vi "PAN_RunMacro.vi"(8 "error in (no error)":errorcluster, 10 "commands":string, 11 "macrodir":path) -> (0 "error out":errorcluster, 2 "response":string)   [LabVIEW 2016]
panel:
  in  "type specifier VI Refnum (for type only)":refnum<vi>
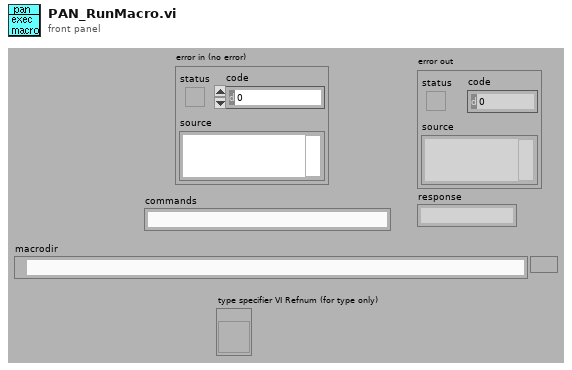
[diagram p1: front panel]
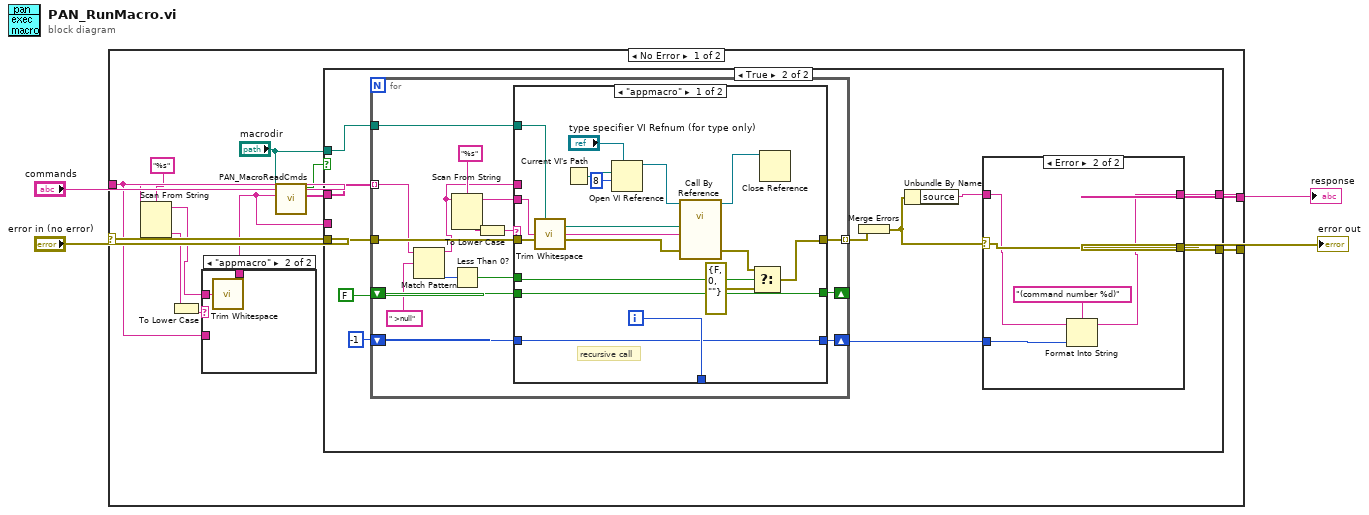
[diagram p0: block diagram]
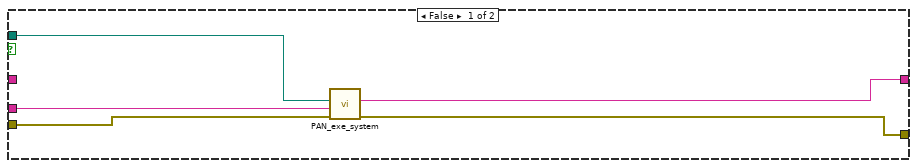
[diagram p3: hidden frame]
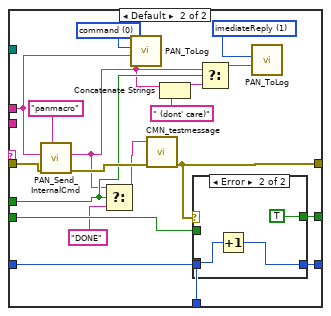
[diagram p5: hidden frame]
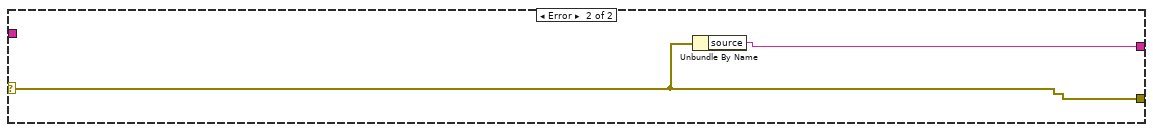
[diagram p7: hidden frame]
diagram:
  n1 = case shown="No Error" "error in (no error)" {
    selector: "error in (no error)" -> [w16 w99]
    tunnel: "commands" -> [w6 _]
    tunnel: [w14 w99] -> w3
    tunnel: [w15 w100] -> w2
    frame No Error {
      n2 = Scan From String(format string="%s", input string=w6) -> (remaining string=w7:string, output 1=w9:string)  [unwired: 2 in, 3 out]
      n3 = To Lower Case(string=w9) -> (all lower case string=w8:string)
      n4 = case shown="\"appmacro\"" w8 {
        tunnel: w7 -> [_ w19]
        tunnel: w6 -> [w17 _]
        tunnel: [w17 w18] -> w5
        frame Default {
        }
        frame "appmacro" {
          n5 = call <vilib>:"Trim Whitespace.vi"("string"=w19) -> ("trimmed string"=w18:string)  [unwired: 1 in]
        }
      }
      n6 = call "PAN_MacroReadCmds.vi"("CommandStr"=w5, "macrodir"="macrodir") -> ("commands"=w13:string[], "macro"=w12:bool)  [unwired: 8 out]
      n7 = case shown="True" w12 {
        tunnel: w16 -> [w22 w34]
        tunnel: [w21 w31] -> w15
        tunnel: [w20 w30] -> w14
        tunnel: w13 -> [_ w26]
        tunnel: "macrodir" -> [w24 w25]
        tunnel: w5 -> [w23 _]
        frame False {
          n8 = call "PAN_exe_system.vi"("error in (no error)"=w22, "command line"=w23, "working directory"=w24) -> ("error out"=w20:errorcluster, "response"=w21:string)  [unwired: 1 in, 6 out]
        }
        frame True {
          n9 = for {
            tunnel: w26 -> [w44] mode=indexing
            tunnel: [w56] -> w35 mode=indexing
            tunnel: w34 -> [w59]
            shift-right: [w54] -> _
            shift-left: FALSE -> [w53]
            shift-right: [w55] -> w27
            shift-left: -1 ("f") -> [w57]
            tunnel: w25 -> [w49]
            i -> [w58]
            n10 = Match Pattern(string=w44, regular expression=" >null") -> (before substring=w43:string, offset past match=w46:i32)  [unwired: 3 out]
            n11 = Scan From String(format string="%s", input string=w43) -> (remaining string=w48:string, output 1=w51:string)  [unwired: 2 in, 3 out]
            n12 = Less Than 0?(x=w46) -> (x < 0?=w45:bool)
            n13 = To Lower Case(string=w51) -> (all lower case string=w50:string)
            n14 = case shown="\"appmacro\"" w50 {
              tunnel: w59 -> [w69 w93]
              tunnel: w58 -> [_ w92]
              tunnel: w57 -> [w74 w91]
              tunnel: [w61 w90] -> w56
              tunnel: [w74 w89] -> w55
              tunnel: [w73 w88] -> w54
              tunnel: w53 -> [w73 w87]
              tunnel: w43 -> [_ w82]
              tunnel: w49 -> [w70 _]
              tunnel: w48 -> [w66 _]
              tunnel: w45 -> [w63 w79]
              frame "appmacro" {
                # "recursive call"
                n15 = call <vilib>:"Trim Whitespace.vi"("string"=w66) -> ("trimmed string"=w67:string)  [unwired: 1 in]
                n16 = Current VI's Path() -> (path=w68:path)
                n17 = Open VI Reference(type specifier VI Refnum (for type only)="type specifier VI Refnum (for type only)", vi path=w68, options=8) -> (vi reference=w71:refnum<vi>)  [unwired: 1 in, 3 out]
                n18 = call-by-ref "?"(reference=w71, "error in"=w69, "CommandStr"=w67, "macrodir"=w70) -> (reference out=w65:refnum<vi>, "error out"=w62:errorcluster)  [unwired: 8 in, 2 out]
                n19 = Select(t=w62, s=w63, f=errorcluster {"status"=FALSE, "code"=0, "source"=""}) -> (s? t:f=w61:errorcluster)
                n20 = Close Reference(reference=w65) -> ()  [unwired: 1 in, 1 out]
              }
              frame Default {
                w84 = u16 1 items=["command", "imediateReply", "Callback Reply", "Information"] ("type")
                w85 = u16 0 items=["command", "imediateReply", "Callback Reply", "Information"] ("type")
                n21 = call "PAN_Send_InternalCmd.vi"("taskID"="panmacro", "error in (no error)"=w93, "command"=w82) -> ("error out"=w86:errorcluster, "response"=w78:string)  [unwired: 2 in, 5 out]
                n22 = Select(t=w78, s=w79, f="DONE") -> (s? t:f=w81:string)
                n23 = call "PAN_ToLog.vi"("message"=w82, "type"=w85) -> ()  [unwired: 2 in, 8 out]
                n24 = call "CMN_testmessage.vi"("error in (no error)"=w86, "message  in"=w81) -> ("error out"=w90:errorcluster)  [unwired: 9 out]
                n25 = Concatenate Strings(w78, " (dont' care)" ("string")) -> (w76:string)
                n26 = case shown="Error" w90 {
                  tunnel: w92 -> [_ w97]
                  tunnel: w91 -> [w95 _]
                  tunnel: [w95 w96] -> w89
                  tunnel: [w94 TRUE] -> w88
                  tunnel: w87 -> [w94 _]
                  frame No Error {
                  }
                  frame Error {
                    n27 = Increment(x=w97) -> (x+1=w96:i32)
                  }
                }
                n28 = Select(t=w78, s=w79, f=w76) -> (s? t:f=w75:string)
                n29 = call "PAN_ToLog.vi"("message"=w75, "type"=w84) -> ()  [unwired: 2 in, 8 out]
              }
            }
          }
          n30 = Merge Errors(w35) -> (w33:errorcluster)
          n31 = Unbundle By Name(w33) -> ("source"=w32:string)
          n32 = case shown="Error" w33 {
            selector: w33 -> [w36 w42]
            tunnel: w32 -> [w37 w39]
            tunnel: [w37 w38] -> w31
            tunnel: [w36 w42] -> w30
            tunnel: w27 -> [_ w40]
            frame No Error {
            }
            frame Error {
              n33 = Format Into String(format string="(command number %d)", initial string=w39, w40) -> (resulting string=w38:string)  [unwired: 1 in, 1 out]
            }
          }
        }
      }
    }
    frame Error {
      n34 = Unbundle By Name(w99) -> ("source"=w100:string)
    }
  }
  "error out" <- w3
  "response" <- w2
